vi "Timer_Start_Internal.vi"(8 "FPGA_Time_Seconds":dbl, 11 "in Timer in":T1 {"Accumulated TIme" format="%13.5p"; "StartTime" format="%13.5p"}) -> (3 "in Timer out":T1 {"Accumulated TIme" format="%13.5p"; "StartTime" format="%13.5p"})   [LabVIEW 2019, in "Trajectory_Library.lvlib"]
doc: "Start Timer Internal -- This is a priviate internal routine. It should NEVER be called by users.\n\nInput:\n -- in Timer -- data cluster\n -- PassThroughTime -- fpga time\n\nOutput\n -- out Timer -- data cluster"
uses:
  Trajectory_Library.lvlib
  TypeDef/TIMER.ctl
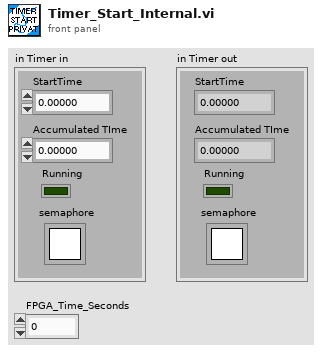
[diagram p1: front panel]
types:
  T1 = typedef "Trajectory_Library.lvlib/TIMER.ctl" = cluster{"StartTime":dbl, "Accumulated TIme":dbl, "Running":bool, "semaphore":T2}
  T2 = typedef "Semaphore RefNum" = refnum<k1>
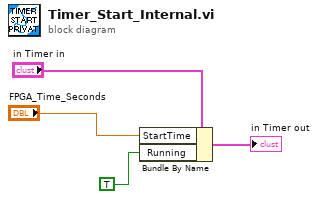
[diagram p0: block diagram]
diagram:
  n1 = Bundle By Name(cluster="in Timer in", "StartTime"="FPGA_Time_Seconds", "Running"=TRUE) -> (→"in Timer out":T1)
